vi "BackProp.vi"(0 "Current Layer":dbl[](array[numeric]), 5 "Previous Layer":dbl[](array[numeric]), 9 "weights":dbl[](array[numeric]), 11 "PreviousWeights":dbl[](array[numeric]), 13 "Target":dbl[](array[numeric])) -> (4 "w+":dbl[](array[numeric]), 6 "dE_dNET":dbl[](array[numeric]))   [LabVIEW 2014]
panel:
  out "dE_dWi":dbl[](array[numeric])
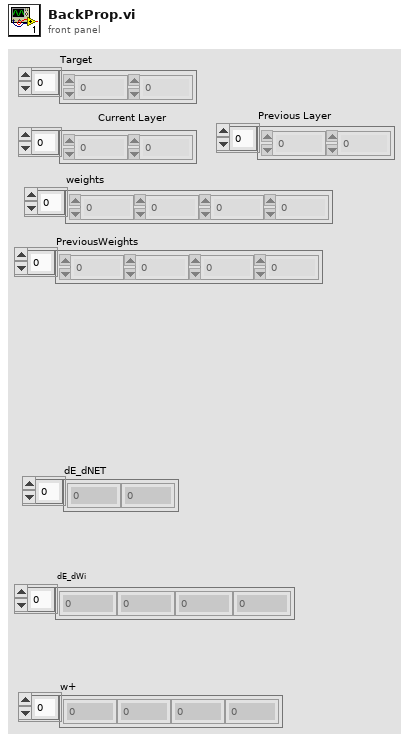
[diagram p1: front panel]
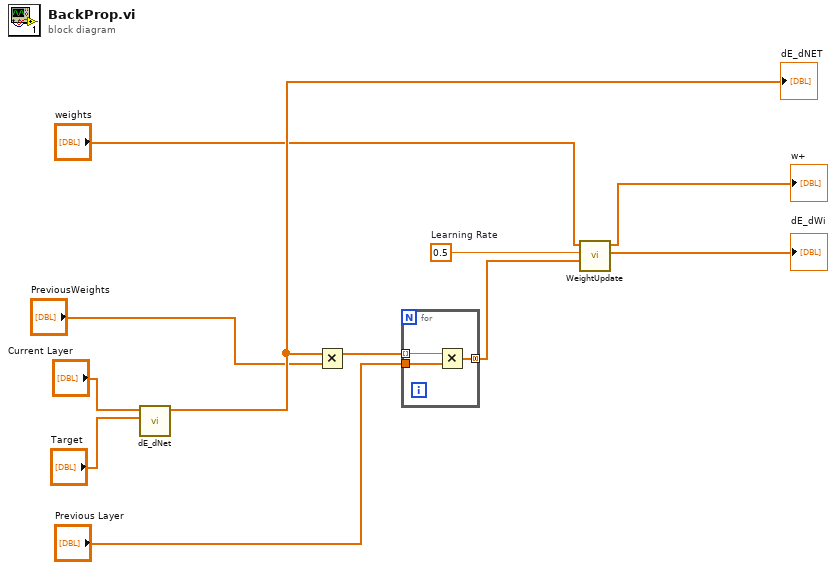
[diagram p0: block diagram]
diagram:
  w10 = 0.5  # Learning Rate
  n1 = call "dE_dNet.vi"("Target"="Target", "Curren Layer OP"="Current Layer") -> ("dE/dNet"=w11:dbl[])  [unwired: 9 in]
  "dE_dNET" <- w11
  n2 = Multiply(x=w11, y="PreviousWeights") -> (x*y=w2:dbl[])
  n3 = for {
    tunnel: w2 -> [w14] mode=indexing
    tunnel: "Previous Layer" -> [w13]
    tunnel: [w12] -> w6 mode=concatenating
    n4 = Multiply(x=w14, y=w13) -> (x*y=w12:dbl[])
  }
  n5 = call "WeightUpdate.vi"("(dE/dOut)(PrevLayerOP)"=w6, "Learning Rate"=w10, "weights"="weights") -> ("dE/dWi"=→"dE_dWi":dbl[], "w+"=→"w+":dbl[])  [unwired: 7 in]
